vi "MyTopic ComplexType Writer.vi"(10 "Parameters":variant, 11 "Process":refnum<class "Process.lvclass">) -> ()   [LabVIEW 2016, in "DDS Custom Device Engine.lvlib"]
uses:
  DDS Custom Device Engine.lvlib
  Shared/MyTopic ComplexType.ctl
  <vilib>/ni/NIVS Inline Async API/_VS Inline Async API/Process/Process.lvclass
  Shared/WriterReaderConfiguration.ctl
  Shared/Advanced DDS Configuration.ctl
  Shared/key Enum.ctl
  <vilib>/RTI DDS Toolkit/Types/RTI DDS ContentFilteredTopic Info.ctl
  <vilib>/ni/NIVS Inline Async API/_VS Inline Async API/Process/Process.lvclass/Process.ctl
  <vilib>/ni/NIVS Inline Async API/_Data Access Engine/Access Type Classes/Read/Read.lvclass/Read.ctl
  <vilib>/ni/NIVS Inline Async API/_Data Access Engine/Data Access Engine/Methods/Read.Data.vi
  <vilib>/ni/NIVS Inline Async API/_VS Inline Async API/Process/Data Member Access/Read Data Access.vi
  <vilib>/ni/NIVS Inline Async API/_VS Inline Async API/Error Handling Process/SubVIs/Error.ConvertArray.vi
  <vilib>/ni/NIVS Inline Async API/_Data Access Engine/Access Type Classes/Read/Read.ProcessData.vi
  <vilib>/ni/NIVS Inline Async API/_Data Access Engine/Data Access Engine/Methods/Read.Lookup.vi
  <vilib>/ni/NIVS Inline Async API/_Data Access Engine/Data Access Engine/Data Access Engine.lvclass
  <vilib>/RTI DDS Toolkit/Library/LVDDS_library.lvlib
  Shared/DDS Custom Device Shared.lvlib
panel:
  in  "MyComplexType type":T1={"I32_Num"=0, "I64_Num"=0, "U16_Num"=0, "Sgl_Array"=[1.0, 1.0, 1.0, 1.0], "innercluster"={"Sgl_Num"=0.0, "Boolean"=FALSE}}
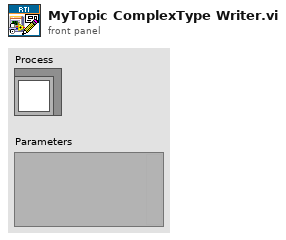
[diagram p1: front panel]
types:
  T1 = typedef "DDS Custom Device Shared.lvlib/MyTopic ComplexType.ctl" = cluster{"I32_Num":i32, "I64_Num":i64, "U16_Num":u16, "Sgl_Array":sgl[], "innercluster":cluster{"Sgl_Num":sgl, "Boolean":bool}}
  T2 = typedef "DDS Custom Device Shared.lvlib/WriterReaderConfiguration.ctl" = cluster{"Topic Name":string, "Domain Id":u32, "Advanced Configuration":T3}
  T3 = typedef "DDS Custom Device Shared.lvlib/Advanced DDS Configuration.ctl" = cluster{"typeName":string, "key Name":T4, "domainParticipantQoSProfile":string, "dataWriterQoSProfile":string, "forceArrayMapping?":bool, "forceUnboundedString?":bool, "forceExclusiveReader?":bool, "forceRead? (only ExclusiveReader)":bool, "ContentFilteredTopic Info":T5}
  T4 = typedef "DDS Custom Device Shared.lvlib/key Enum.ctl" = enum16{"<none>", "I32_Num", "I64_Num", "U16_Num", "innercluster.Sgl_Num", "innercluster.Boolean"}
  T5 = typedef "LVDDS_library.lvlib/RTI DDS ContentFilteredTopic Info.ctl" = cluster{"Filter Type":string, "ContentFilteredTopic Name":string, "Filter Expression":string}
  T6 = typedef "Data Access Engine.lvlib/Data Access Engine.lvclass/Read.DVR.ctl" = refnum<data-value>
  T7 = typedef "LVDDS_library.lvlib/RTI DDS Advanced Writer Configuration.ctl" = cluster{"typeName":string, "keyName":string, "domainParticipantQoSProfile":string, "dataWriterQoSProfile":string, "forceArrayMapping?":bool, "forceUnboundedString?":bool}
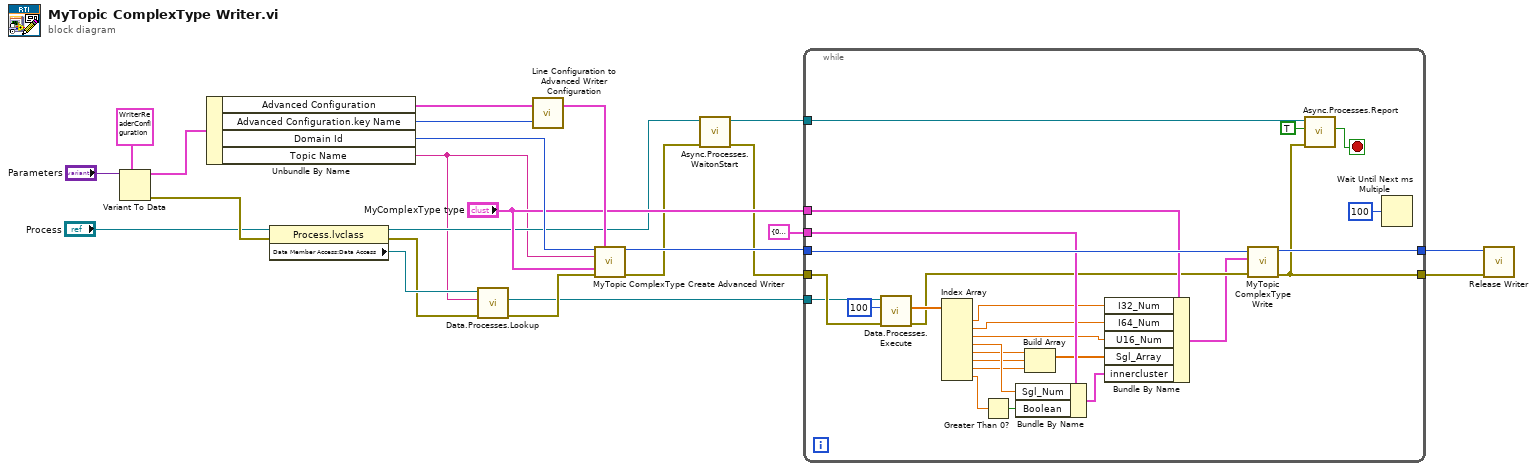
[diagram p0: block diagram]
diagram:
  n1 = Variant To Data(type=T2 {"Topic Name"="MyTopic", "Domain Id"=0, "Advanced Configuration"={"typeName"="", "key Name"=enum."<none>", "domainParticipantQoSProfile"="", "dataWriterQoSProfile"="", "forceArrayMapping?"=FALSE, "forceUnboundedString?"=FALSE, "forceExclusiveReader?"=FALSE, "forceRead? (only ExclusiveReader)"=FALSE, "ContentFilteredTopic Info"={"Filter Type"="DDS_SQLFILTER_NAME", "ContentFilteredTopic Name"="", "Filter Expression"=""}}} ("Line"), Variant="Parameters") -> (data=w16:T2, error out=w17:errorcluster)  [unwired: 1 in]
  n2 = Unbundle By Name(w16) -> ("Advanced Configuration"=w2:T3, "Advanced Configuration.key Name"=w3:T4, "Domain Id"=w14:u32, "Topic Name"=w1:string)
  n3 = property class="Process.lvclass"(reference="Process", error in=w17) -> (reference out=w8:refnum<class "Process.lvclass">, error out=w19:errorcluster, "Data Member Access:Data Access"=w21:refnum<class "Data Access Engine.lvclass">)
  n4 = call-poly <vilib>:"Data.Processes.Lookup.vi"("error in (no error)"=w19, "Name"=w1, "Data Access API in"=w21) -> ("error out"=w13:errorcluster, "Ref"=w12:T6)  [unwired: 5 in, 2 out]
  n5 = call "Line Configuration to Advanced Writer Configuration.vi"("key Name"=w3, "Advanced Configuration"=w2) -> ("Advanced Writer Configuration"=w15:T7)  [unwired: 1 in]
  n6 = call "MyTopic ComplexType Create Advanced Writer.vi"("Domain Id"=w14, "Advanced Writer Configuration"=w15, "Topic Name"=w1, "MyComplexType type"="MyComplexType type", "error in (no error)"=w13) -> ("Refnum"=w22:u64, "error out"=w7:errorcluster)  [unwired: 9 in]
  n7 = call <vilib>:"Async.Processes.WaitonStart.vi"("error in (no error)"=w7, "Process"=w8) -> ("error out"=w6:errorcluster, "Process out"=w4:refnum<class "Process.lvclass">)  [unwired: 7 in, 1 out]
  n8 = while "Main Loop" {
    tunnel: w22 -> [w49]
    tunnel: [w47] -> w23
    tunnel: w6 -> [w46]
    tunnel: w12 -> [w45]
    tunnel: "MyComplexType type" -> [w43]
    tunnel: cluster{"Sgl_Num":sgl, "Boolean":bool} {"Sgl_Num"=0.0, "Boolean"=FALSE} ("innercluster") -> [w42]
    tunnel: [w26] -> w5
    tunnel: w4 -> [w25]
    stop <- w27 stop-if-true
    n9 = call-poly <vilib>:"Data.Processes.Execute.vi"("error in (no error)"=w46, "timeout ms"=100, "Ref"=w45) -> ("error out"=w39:errorcluster, "Values"=w40:dbl[])  [unwired: 6 in, 1 out]
    n10 = Index Array(array=w40) -> (element #1=w38:dbl, element #2=w37:dbl, element #3=w36:dbl, element #4=w34:dbl, element #5=w33:dbl, element #6=w32:dbl, element #7=w31:dbl, element #8=w29:dbl)  [unwired: 8 in]
    n11 = Greater Than 0?(x=w29) -> (x > 0?=w30:bool)
    n12 = Bundle By Name(cluster=w42, "Sgl_Num"=w34, "Boolean"=w30) -> (w41:cluster{"Sgl_Num":sgl, "Boolean":bool})
    n13 = Build Array(w33, w32, w31) -> (w35:dbl[])
    n14 = Bundle By Name(cluster=w43, "I32_Num"=w38, "I64_Num"=w37, "U16_Num"=w36, "Sgl_Array"=w35, "innercluster"=w41) -> (w28:T1)
    n15 = call "MyTopic ComplexType Write.vi"("error in"=w39, "complexType"=w28, "DDS Object Ref"=w49) -> ("error out"=w26:errorcluster, "DDS Object Ref out"=w47:u64)  [unwired: 7 in]
    n16 = call <vilib>:"Async.Processes.Report.vi"("Error"=w26, "Stop Async on Error?"=TRUE, "Process in"=w25) -> ("Stop"=w27:bool)  [unwired: 7 in, 1 out]
    n17 = Wait Until Next ms Multiple(millisecond multiple=u32 100) -> ()  [unwired: 1 out]
  }
  n18 = call <vilib>:"Release Writer.vi"("error in (no error)"=w5, "DDS Object Ref"=w23) -> ()  [unwired: 9 in, 1 out]
